vi "Test parallel sleep.vi"() -> ()   [LabVIEW 2021]
uses:
  <vilib>/Utility/RT CPU Load.ctl
  <vilib>/Platform/TimedLoop/XDataNode/timing_clust.ctl
  <vilib>/Platform/TimedLoop/XDataNode/nitl_modes.ctl
  <vilib>/Platform/TimedLoop/XDataNode/wakeup.ctl
  System Time/LabVIEW Time to TAI Time.vi
  <vilib>/platform/TimedLoop/XDataNode/XDataNode.xnode
  Time_CIF_U.lvlib
  <vilib>/NI_Real-Time Target Support.lvlib
  <vilib>/Platform/TimedLoop/XDataNode/XDNodeRunTimeDep.lvlib
panel:
  out "CPU loads":T1[](array[typedef]) {"ISR (%)" format="%#.2f"; "Idle (%)" format="%#.2f"; "Background (%)" format="%#.2f"; "Normal (%)" format="%#.2f"; "Above Normal (%)" format="%#.2f"; "High (%)" format="%#.2g"; "Timed Structures (%)" format="%#.2g"; "Time Critical (%)" format="%#.2g"; "Total (%)" format="%#.2g"}
  out "appended array":T2(array[cluster])
  in  "stop":bool
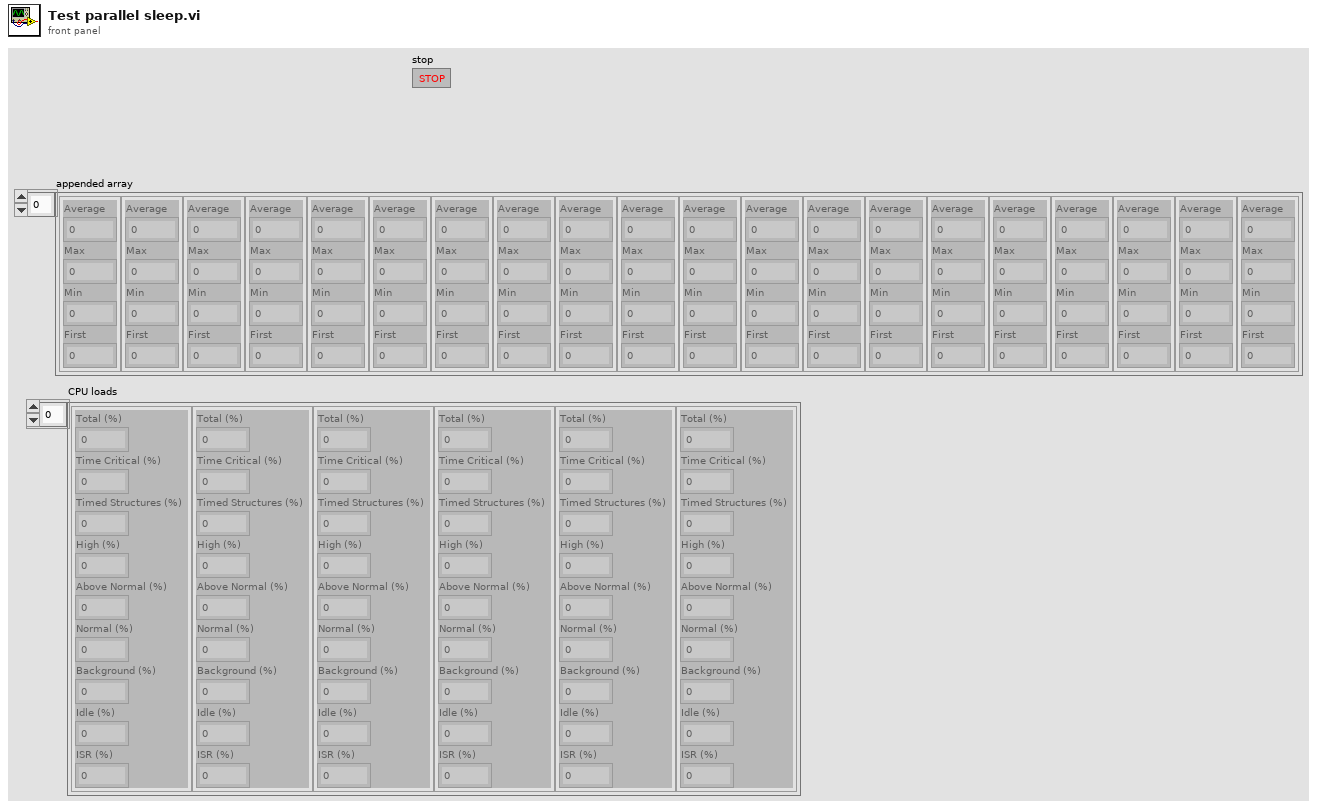
[diagram p1: front panel]
types:
  T1 = typedef "NI_Real-Time Target Support.lvlib/RT CPU Load.ctl" = cluster{"Total (%)":dbl, "Time Critical (%)":dbl, "Timed Structures (%)":dbl, "High (%)":dbl, "Above Normal (%)":dbl, "Normal (%)":dbl, "Background (%)":dbl, "Idle (%)":dbl, "ISR (%)":dbl}
  T2 = cluster{"Average":dbl, "Max":dbl, "Min":dbl, "First":dbl}[]
  T3 = typedef "XDNodeRunTimeDep.lvlib/timing_clust.ctl" = cluster{"Expected End [f-1]":u64, "Actual End [f-1]":u64, "Finished Late? [f-1]":bool, "Expected End [i-1]":u64, "Actual End [i-1]":u64, "Finished Late? [i-1]":bool, "Expected Start [i]":u64, "Actual Start [i]":u64, "Expected Start [f]":u64, "Actual Start [f]":u64, "Source Name":string, "Structure Name":string, "Period":i64, "Deadline":i64, "Offset":i64, "Start":i64, "Priority":i32, "Timeout":i32, "Mode":T4, "Wakeup Reason":T5, "Error":errorcluster, "Source Type":string, "Secondary Source Type":string, "Global End Time":u64, "Global Start Time":u64, "Frame Duration":u64, "Iteration Duration":u64, "Assigned CPU":i32, "I/O Scan Engine Mode":u32}
  T4 = typedef "XDNodeRunTimeDep.lvlib/nitl_modes.ctl" = enum32{"No Change", "Process missed periods, maintain original phase", "Discard missed periods, maintain original phase", "Process missed periods, ignore original phase", "Discard missed periods, ignore original phase"}
  T5 = typedef "XDNodeRunTimeDep.lvlib/wakeup.ctl" = enum32{"Normal", "Aborted", "Asynchronous wakeup", "Timing source error", "Timed loop error", "Timeout"}
  T6 = cluster{"Average":dbl, "Max":dbl, "Min":dbl, "First":dbl}
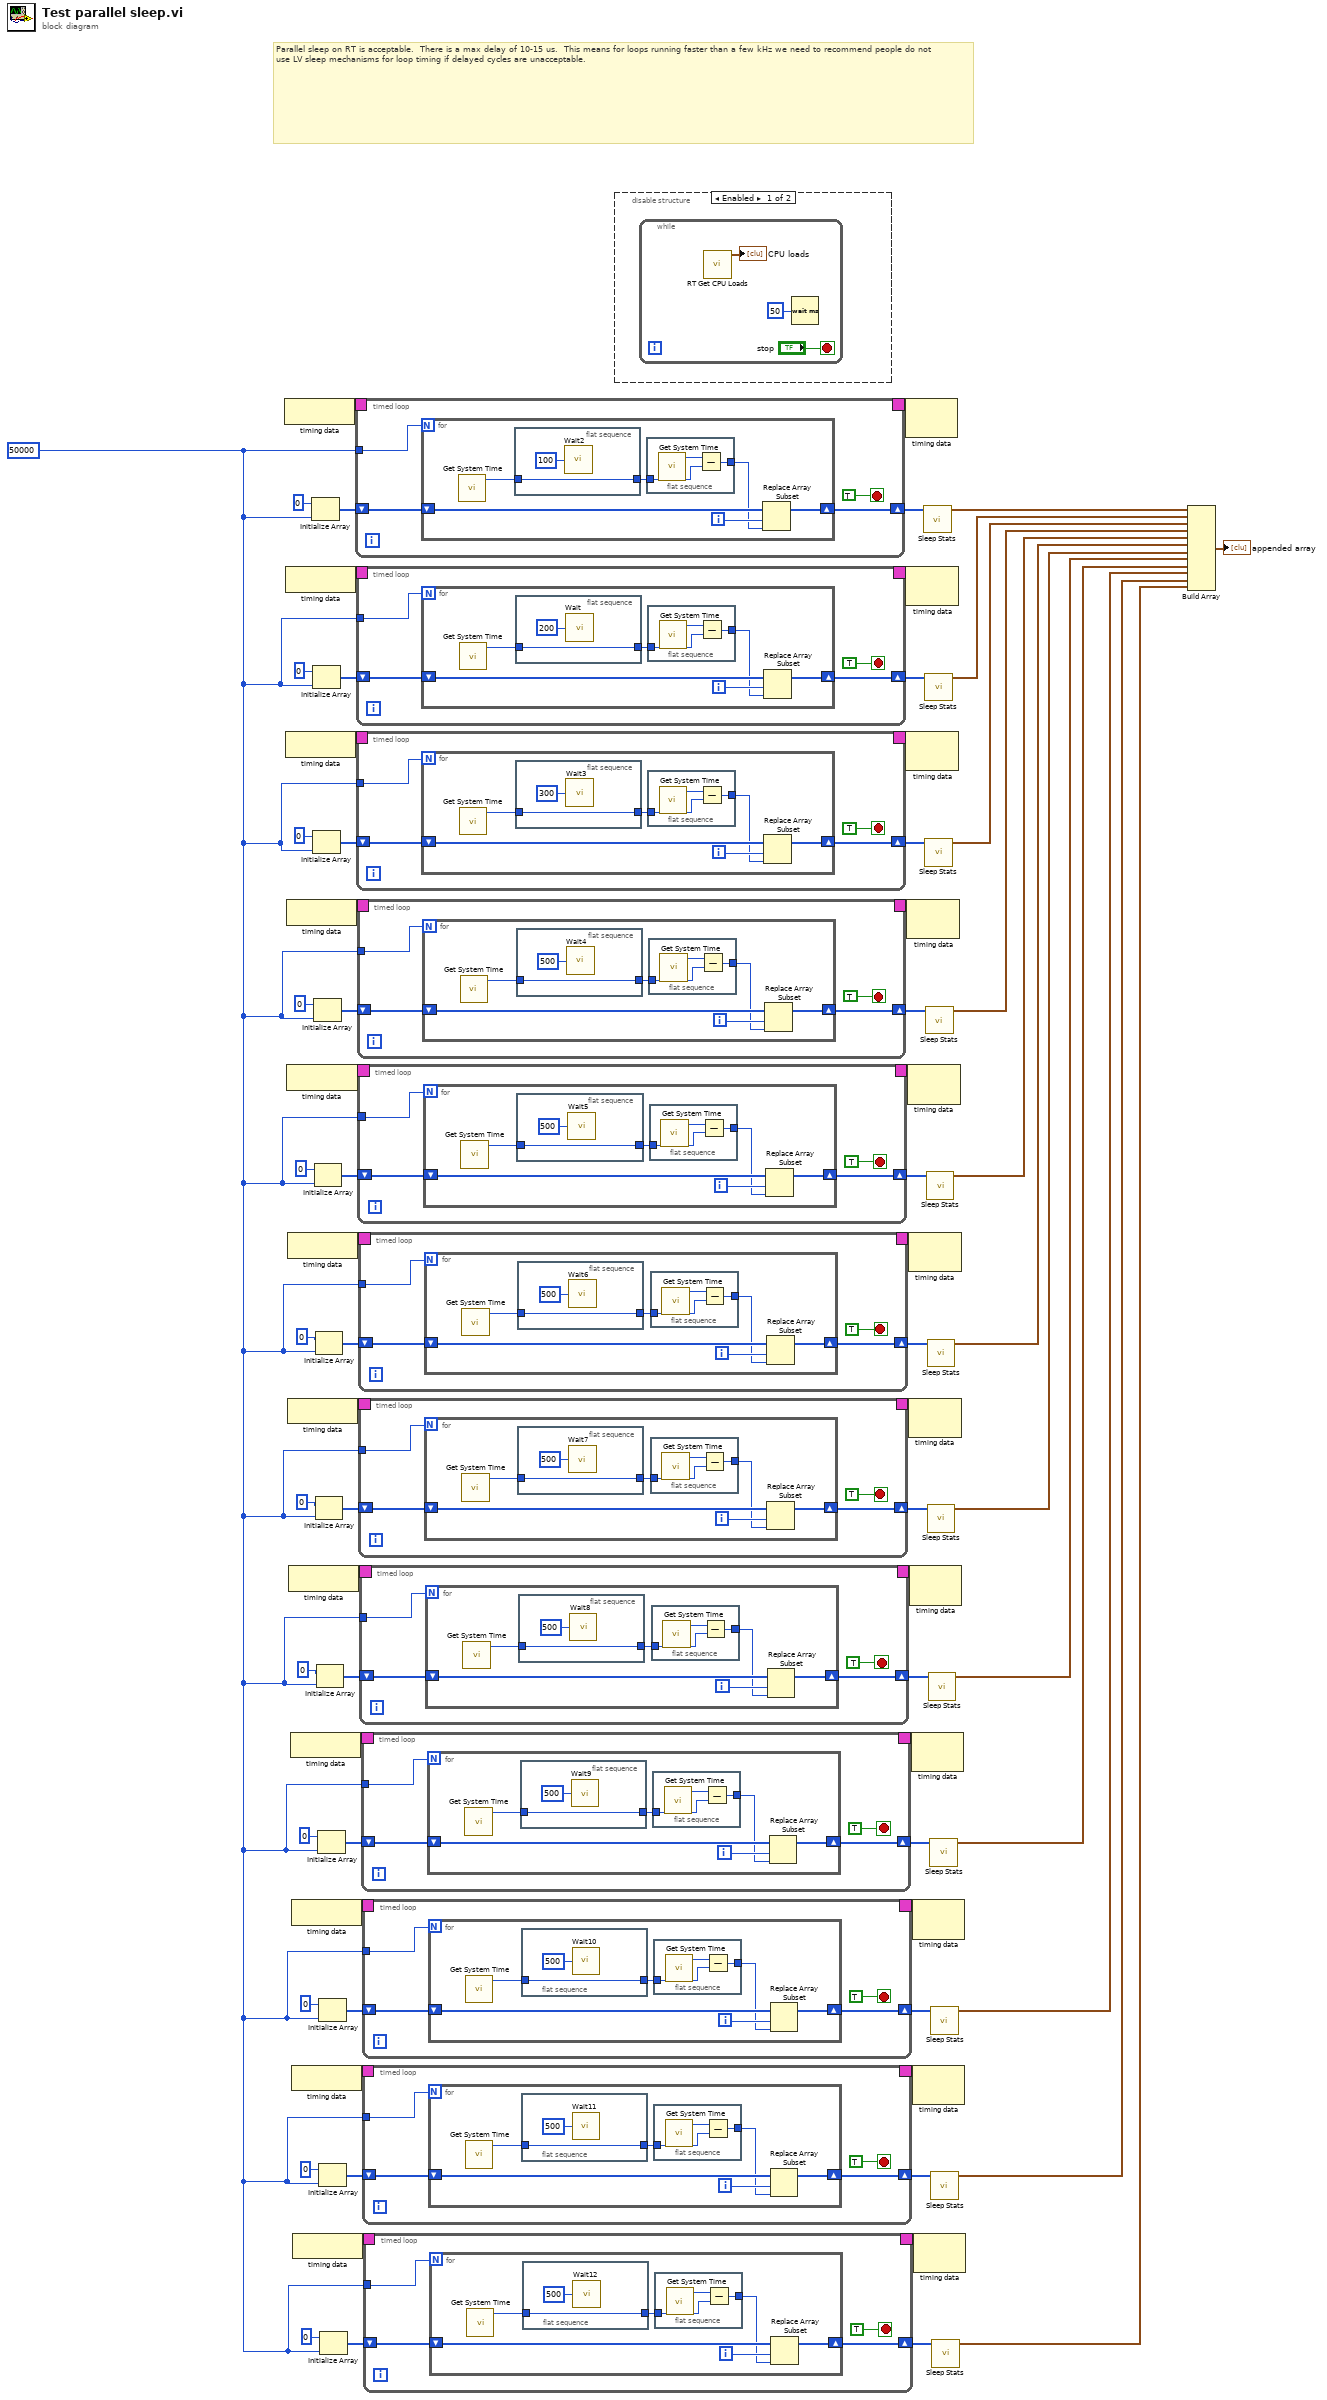
[diagram p0: block diagram]
diagram:
  w1 = 50000
  # "Parallel sleep on RT is acceptable.  There is a max delay of 10-15 us.  This means for loops running faster than a few kHz we need to recommend people do not use LV sleep mechanisms for loop timing if delayed cycles are unacceptable."
  n1 = node-c288() -> (w71:T3)
  n2 = node-c288() -> (w67:T3)
  n3 = node-c288() -> (w62:T3)
  n4 = node-c288() -> (w60:T3)
  n5 = node-c288() -> (w52:T3)
  n6 = node-c288() -> (w50:T3)
  n7 = node-c288() -> (w48:T3)
  n8 = node-c288() -> (w46:T3)
  n9 = node-c288() -> (w32:T3)
  n10 = node-c288() -> (w30:T3)
  n11 = node-c288() -> (w28:T3)
  n12 = node-c288() -> (w26:T3)
  n13 = Initialize Array(u64 0, w1) -> (w73:u64[])
  n14 = Initialize Array(u64 0, w1) -> (w64:u64[])
  n15 = Initialize Array(u64 0, w1) -> (w54:u64[])
  n16 = Initialize Array(u64 0, w1) -> (w57:u64[])
  n17 = Initialize Array(u64 0, w1) -> (w34:u64[])
  n18 = Initialize Array(u64 0, w1) -> (w37:u64[])
  n19 = Initialize Array(u64 0, w1) -> (w43:u64[])
  n20 = Initialize Array(u64 0, w1) -> (w40:u64[])
  n21 = Initialize Array(u64 0, w1) -> (w23:u64[])
  n22 = Initialize Array(u64 0, w1) -> (w20:u64[])
  n23 = Initialize Array(u64 0, w1) -> (w14:u64[])
  n24 = Initialize Array(u64 0, w1) -> (w17:u64[])
  n25 = timed-loop {
    timing: w71 -> [_]
    timing-out: [_] -> w70
    tunnel: w1 -> [w78]
    shift-right: [w76] -> w72
    shift-left: w73 -> [w77]
    stop <- TRUE stop-if-true
    n26 = for {
      N: w78 -> [_]
      shift-right: [w83] -> w76
      shift-left: w77 -> [w84]
      i -> [w82]
      n27 = call "Get System Time.vi"() -> ("Time (ns)"=w80:i64)  [unwired: 5 in]
      n28 = flat-sequence {
        tunnel: w80 -> [w88]
        tunnel: [w88] -> w79
        frame #0 {
          n29 = call "Wait2"("Count(uSec)"=u32 100) -> ()  [unwired: 1 out]
        }
      }
      n30 = flat-sequence {
        tunnel: [w86] -> w81
        tunnel: w79 -> [w85]
        frame #0 {
          n31 = call "Get System Time.vi"() -> ("Time (ns)"=w87:i64)  [unwired: 5 in]
          n32 = Subtract(x=w87, y=w85) -> (x-y=w86:i64)
        }
      }
      n33 = Replace Array Subset(array=w84, new element=w81, index=w82) -> (w83:u64[])
    }
  }
  n34 = timed-loop {
    timing: w67 -> [_]
    timing-out: [_] -> w66
    tunnel: w1 -> [w95]
    shift-right: [w93] -> w65
    shift-left: w64 -> [w94]
    stop <- TRUE stop-if-true
    n35 = for {
      N: w95 -> [_]
      shift-right: [w100] -> w93
      shift-left: w94 -> [w101]
      i -> [w99]
      n36 = call "Get System Time.vi"() -> ("Time (ns)"=w97:i64)  [unwired: 5 in]
      n37 = flat-sequence {
        tunnel: w97 -> [w105]
        tunnel: [w105] -> w96
        frame #0 {
          n38 = call "Wait"("Count(uSec)"=u32 200) -> ()  [unwired: 1 out]
        }
      }
      n39 = flat-sequence {
        tunnel: [w103] -> w98
        tunnel: w96 -> [w102]
        frame #0 {
          n40 = call "Get System Time.vi"() -> ("Time (ns)"=w104:i64)  [unwired: 5 in]
          n41 = Subtract(x=w104, y=w102) -> (x-y=w103:i64)
        }
      }
      n42 = Replace Array Subset(array=w101, new element=w98, index=w99) -> (w100:u64[])
    }
  }
  n43 = timed-loop {
    timing: w62 -> [_]
    timing-out: [_] -> w61
    tunnel: w1 -> [w112]
    shift-right: [w110] -> w55
    shift-left: w54 -> [w111]
    stop <- TRUE stop-if-true
    n44 = for {
      N: w112 -> [_]
      shift-right: [w117] -> w110
      shift-left: w111 -> [w118]
      i -> [w116]
      n45 = call "Get System Time.vi"() -> ("Time (ns)"=w114:i64)  [unwired: 5 in]
      n46 = flat-sequence {
        tunnel: w114 -> [w122]
        tunnel: [w122] -> w113
        frame #0 {
          n47 = call "Wait3"("Count(uSec)"=u32 300) -> ()  [unwired: 1 out]
        }
      }
      n48 = flat-sequence {
        tunnel: [w120] -> w115
        tunnel: w113 -> [w119]
        frame #0 {
          n49 = call "Get System Time.vi"() -> ("Time (ns)"=w121:i64)  [unwired: 5 in]
          n50 = Subtract(x=w121, y=w119) -> (x-y=w120:i64)
        }
      }
      n51 = Replace Array Subset(array=w118, new element=w115, index=w116) -> (w117:u64[])
    }
  }
  n52 = timed-loop {
    timing: w60 -> [_]
    timing-out: [_] -> w59
    tunnel: w1 -> [w129]
    shift-right: [w127] -> w56
    shift-left: w57 -> [w128]
    stop <- TRUE stop-if-true
    n53 = for {
      N: w129 -> [_]
      shift-right: [w134] -> w127
      shift-left: w128 -> [w135]
      i -> [w133]
      n54 = call "Get System Time.vi"() -> ("Time (ns)"=w131:i64)  [unwired: 5 in]
      n55 = flat-sequence {
        tunnel: w131 -> [w139]
        tunnel: [w139] -> w130
        frame #0 {
          n56 = call "Wait4"("Count(uSec)"=u32 500) -> ()  [unwired: 1 out]
        }
      }
      n57 = flat-sequence {
        tunnel: [w137] -> w132
        tunnel: w130 -> [w136]
        frame #0 {
          n58 = call "Get System Time.vi"() -> ("Time (ns)"=w138:i64)  [unwired: 5 in]
          n59 = Subtract(x=w138, y=w136) -> (x-y=w137:i64)
        }
      }
      n60 = Replace Array Subset(array=w135, new element=w132, index=w133) -> (w134:u64[])
    }
  }
  n61 = timed-loop {
    timing: w52 -> [_]
    timing-out: [_] -> w51
    tunnel: w1 -> [w146]
    shift-right: [w144] -> w35
    shift-left: w34 -> [w145]
    stop <- TRUE stop-if-true
    n62 = for {
      N: w146 -> [_]
      shift-right: [w151] -> w144
      shift-left: w145 -> [w152]
      i -> [w150]
      n63 = call "Get System Time.vi"() -> ("Time (ns)"=w148:i64)  [unwired: 5 in]
      n64 = flat-sequence {
        tunnel: w148 -> [w156]
        tunnel: [w156] -> w147
        frame #0 {
          n65 = call "Wait5"("Count(uSec)"=u32 500) -> ()  [unwired: 1 out]
        }
      }
      n66 = flat-sequence {
        tunnel: [w154] -> w149
        tunnel: w147 -> [w153]
        frame #0 {
          n67 = call "Get System Time.vi"() -> ("Time (ns)"=w155:i64)  [unwired: 5 in]
          n68 = Subtract(x=w155, y=w153) -> (x-y=w154:i64)
        }
      }
      n69 = Replace Array Subset(array=w152, new element=w149, index=w150) -> (w151:u64[])
    }
  }
  n70 = timed-loop {
    timing: w50 -> [_]
    timing-out: [_] -> w49
    tunnel: w1 -> [w163]
    shift-right: [w161] -> w36
    shift-left: w37 -> [w162]
    stop <- TRUE stop-if-true
    n71 = for {
      N: w163 -> [_]
      shift-right: [w168] -> w161
      shift-left: w162 -> [w169]
      i -> [w167]
      n72 = call "Get System Time.vi"() -> ("Time (ns)"=w165:i64)  [unwired: 5 in]
      n73 = flat-sequence {
        tunnel: w165 -> [w173]
        tunnel: [w173] -> w164
        frame #0 {
          n74 = call "Wait6"("Count(uSec)"=u32 500) -> ()  [unwired: 1 out]
        }
      }
      n75 = flat-sequence {
        tunnel: [w171] -> w166
        tunnel: w164 -> [w170]
        frame #0 {
          n76 = call "Get System Time.vi"() -> ("Time (ns)"=w172:i64)  [unwired: 5 in]
          n77 = Subtract(x=w172, y=w170) -> (x-y=w171:i64)
        }
      }
      n78 = Replace Array Subset(array=w169, new element=w166, index=w167) -> (w168:u64[])
    }
  }
  n79 = timed-loop {
    timing: w48 -> [_]
    timing-out: [_] -> w47
    tunnel: w1 -> [w180]
    shift-right: [w178] -> w42
    shift-left: w43 -> [w179]
    stop <- TRUE stop-if-true
    n80 = for {
      N: w180 -> [_]
      shift-right: [w185] -> w178
      shift-left: w179 -> [w186]
      i -> [w184]
      n81 = call "Get System Time.vi"() -> ("Time (ns)"=w182:i64)  [unwired: 5 in]
      n82 = flat-sequence {
        tunnel: w182 -> [w190]
        tunnel: [w190] -> w181
        frame #0 {
          n83 = call "Wait7"("Count(uSec)"=u32 500) -> ()  [unwired: 1 out]
        }
      }
      n84 = flat-sequence {
        tunnel: [w188] -> w183
        tunnel: w181 -> [w187]
        frame #0 {
          n85 = call "Get System Time.vi"() -> ("Time (ns)"=w189:i64)  [unwired: 5 in]
          n86 = Subtract(x=w189, y=w187) -> (x-y=w188:i64)
        }
      }
      n87 = Replace Array Subset(array=w186, new element=w183, index=w184) -> (w185:u64[])
    }
  }
  n88 = timed-loop {
    timing: w46 -> [_]
    timing-out: [_] -> w45
    tunnel: w1 -> [w197]
    shift-right: [w195] -> w41
    shift-left: w40 -> [w196]
    stop <- TRUE stop-if-true
    n89 = for {
      N: w197 -> [_]
      shift-right: [w202] -> w195
      shift-left: w196 -> [w203]
      i -> [w201]
      n90 = call "Get System Time.vi"() -> ("Time (ns)"=w199:i64)  [unwired: 5 in]
      n91 = flat-sequence {
        tunnel: w199 -> [w207]
        tunnel: [w207] -> w198
        frame #0 {
          n92 = call "Wait8"("Count(uSec)"=u32 500) -> ()  [unwired: 1 out]
        }
      }
      n93 = flat-sequence {
        tunnel: [w205] -> w200
        tunnel: w198 -> [w204]
        frame #0 {
          n94 = call "Get System Time.vi"() -> ("Time (ns)"=w206:i64)  [unwired: 5 in]
          n95 = Subtract(x=w206, y=w204) -> (x-y=w205:i64)
        }
      }
      n96 = Replace Array Subset(array=w203, new element=w200, index=w201) -> (w202:u64[])
    }
  }
  n97 = timed-loop {
    timing: w32 -> [_]
    timing-out: [_] -> w31
    tunnel: w1 -> [w214]
    shift-right: [w212] -> w22
    shift-left: w23 -> [w213]
    stop <- TRUE stop-if-true
    n98 = for {
      N: w214 -> [_]
      shift-right: [w219] -> w212
      shift-left: w213 -> [w220]
      i -> [w218]
      n99 = call "Get System Time.vi"() -> ("Time (ns)"=w216:i64)  [unwired: 5 in]
      n100 = flat-sequence {
        tunnel: w216 -> [w224]
        tunnel: [w224] -> w215
        frame #0 {
          n101 = call "Wait9"("Count(uSec)"=u32 500) -> ()  [unwired: 1 out]
        }
      }
      n102 = flat-sequence {
        tunnel: [w222] -> w217
        tunnel: w215 -> [w221]
        frame #0 {
          n103 = call "Get System Time.vi"() -> ("Time (ns)"=w223:i64)  [unwired: 5 in]
          n104 = Subtract(x=w223, y=w221) -> (x-y=w222:i64)
        }
      }
      n105 = Replace Array Subset(array=w220, new element=w217, index=w218) -> (w219:u64[])
    }
  }
  n106 = timed-loop {
    timing: w30 -> [_]
    timing-out: [_] -> w29
    tunnel: w1 -> [w231]
    shift-right: [w229] -> w21
    shift-left: w20 -> [w230]
    stop <- TRUE stop-if-true
    n107 = for {
      N: w231 -> [_]
      shift-right: [w236] -> w229
      shift-left: w230 -> [w237]
      i -> [w235]
      n108 = call "Get System Time.vi"() -> ("Time (ns)"=w233:i64)  [unwired: 5 in]
      n109 = flat-sequence {
        tunnel: w233 -> [w241]
        tunnel: [w241] -> w232
        frame #0 {
          n110 = call "Wait10"("Count(uSec)"=u32 500) -> ()  [unwired: 1 out]
        }
      }
      n111 = flat-sequence {
        tunnel: [w239] -> w234
        tunnel: w232 -> [w238]
        frame #0 {
          n112 = call "Get System Time.vi"() -> ("Time (ns)"=w240:i64)  [unwired: 5 in]
          n113 = Subtract(x=w240, y=w238) -> (x-y=w239:i64)
        }
      }
      n114 = Replace Array Subset(array=w237, new element=w234, index=w235) -> (w236:u64[])
    }
  }
  n115 = timed-loop {
    timing: w28 -> [_]
    timing-out: [_] -> w27
    tunnel: w1 -> [w248]
    shift-right: [w246] -> w15
    shift-left: w14 -> [w247]
    stop <- TRUE stop-if-true
    n116 = for {
      N: w248 -> [_]
      shift-right: [w253] -> w246
      shift-left: w247 -> [w254]
      i -> [w252]
      n117 = call "Get System Time.vi"() -> ("Time (ns)"=w250:i64)  [unwired: 5 in]
      n118 = flat-sequence {
        tunnel: w250 -> [w258]
        tunnel: [w258] -> w249
        frame #0 {
          n119 = call "Wait11"("Count(uSec)"=u32 500) -> ()  [unwired: 1 out]
        }
      }
      n120 = flat-sequence {
        tunnel: [w256] -> w251
        tunnel: w249 -> [w255]
        frame #0 {
          n121 = call "Get System Time.vi"() -> ("Time (ns)"=w257:i64)  [unwired: 5 in]
          n122 = Subtract(x=w257, y=w255) -> (x-y=w256:i64)
        }
      }
      n123 = Replace Array Subset(array=w254, new element=w251, index=w252) -> (w253:u64[])
    }
  }
  n124 = timed-loop {
    timing: w26 -> [_]
    timing-out: [_] -> w25
    tunnel: w1 -> [w265]
    shift-right: [w263] -> w16
    shift-left: w17 -> [w264]
    stop <- TRUE stop-if-true
    n125 = for {
      N: w265 -> [_]
      shift-right: [w270] -> w263
      shift-left: w264 -> [w271]
      i -> [w269]
      n126 = call "Get System Time.vi"() -> ("Time (ns)"=w267:i64)  [unwired: 5 in]
      n127 = flat-sequence {
        tunnel: w267 -> [w275]
        tunnel: [w275] -> w266
        frame #0 {
          n128 = call "Wait12"("Count(uSec)"=u32 500) -> ()  [unwired: 1 out]
        }
      }
      n129 = flat-sequence {
        tunnel: [w273] -> w268
        tunnel: w266 -> [w272]
        frame #0 {
          n130 = call "Get System Time.vi"() -> ("Time (ns)"=w274:i64)  [unwired: 5 in]
          n131 = Subtract(x=w274, y=w272) -> (x-y=w273:i64)
        }
      }
      n132 = Replace Array Subset(array=w271, new element=w268, index=w269) -> (w270:u64[])
    }
  }
  n133 = disable-structure shown="Enabled" {
    frame Enabled {
      n134 = while {
        stop <- "stop" stop-if-true
        n135 = call <vilib>:"RT Get CPU Loads.vi"() -> ("CPU loads"=→"CPU loads":T1[])  [unwired: 10 in, 1 out]
        n136 = Wait (ms)(milliseconds to wait=u32 50) -> ()  [unwired: 1 out]
      }
    }
    frame Disabled {
    }
  }
  n137 = node-c288(w70) -> ()  [unwired: 1 out]
  n138 = node-c288(w66) -> ()  [unwired: 1 out]
  n139 = node-c288(w61) -> ()  [unwired: 1 out]
  n140 = node-c288(w59) -> ()  [unwired: 1 out]
  n141 = node-c288(w51) -> ()  [unwired: 1 out]
  n142 = node-c288(w49) -> ()  [unwired: 1 out]
  n143 = node-c288(w47) -> ()  [unwired: 1 out]
  n144 = node-c288(w45) -> ()  [unwired: 1 out]
  n145 = node-c288(w31) -> ()  [unwired: 1 out]
  n146 = node-c288(w29) -> ()  [unwired: 1 out]
  n147 = node-c288(w27) -> ()  [unwired: 1 out]
  n148 = node-c288(w25) -> ()  [unwired: 1 out]
  n149 = call "Sleep Stats.vi"("Sleep Timers"=w72) -> ("Stats"=w69:T6)  [unwired: 10 in]
  n150 = call "Sleep Stats.vi"("Sleep Timers"=w65) -> ("Stats"=w2:T6)  [unwired: 10 in]
  n151 = call "Sleep Stats.vi"("Sleep Timers"=w55) -> ("Stats"=w3:T6)  [unwired: 10 in]
  n152 = call "Sleep Stats.vi"("Sleep Timers"=w56) -> ("Stats"=w4:T6)  [unwired: 10 in]
  n153 = call "Sleep Stats.vi"("Sleep Timers"=w35) -> ("Stats"=w5:T6)  [unwired: 10 in]
  n154 = call "Sleep Stats.vi"("Sleep Timers"=w36) -> ("Stats"=w6:T6)  [unwired: 10 in]
  n155 = call "Sleep Stats.vi"("Sleep Timers"=w42) -> ("Stats"=w7:T6)  [unwired: 10 in]
  n156 = call "Sleep Stats.vi"("Sleep Timers"=w41) -> ("Stats"=w8:T6)  [unwired: 10 in]
  n157 = call "Sleep Stats.vi"("Sleep Timers"=w22) -> ("Stats"=w9:T6)  [unwired: 10 in]
  n158 = call "Sleep Stats.vi"("Sleep Timers"=w21) -> ("Stats"=w10:T6)  [unwired: 10 in]
  n159 = call "Sleep Stats.vi"("Sleep Timers"=w15) -> ("Stats"=w11:T6)  [unwired: 10 in]
  n160 = call "Sleep Stats.vi"("Sleep Timers"=w16) -> ("Stats"=w12:T6)  [unwired: 10 in]
  n161 = Build Array(w69, w2, w3, w4, w5, w6, w7, w8, w9, w10, w11, w12) -> (→"appended array":T2)
